vi "Flush ByteArray.vi"(8 "error in":errorcluster, 11 "Buffer":refnum<data-value>) -> (0 "error out":errorcluster, 2 "bytes":u8[](array[numeric]) format="%02x", 3 "Buffer":refnum<data-value>)   [LabVIEW 2013, in "ByteBuffer.lvclass"]
doc: "This VI returns data from the ring buffer starting from the oldest data and ending with the newest.\n\nThe data is duplicated at the output so this VI allocates new place in the memory for the output."
uses:
  ByteBuffer.lvclass
  VariantBuffer/VariantBuffer.lvclass
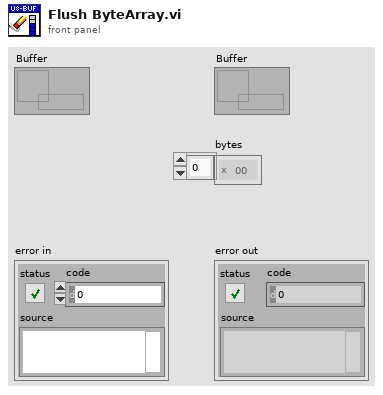
[diagram p1: front panel]
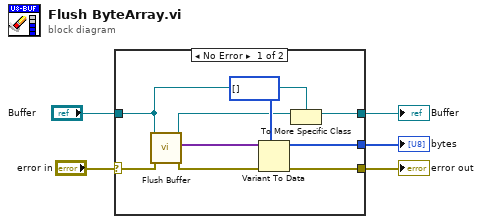
[diagram p0: block diagram]
diagram:
  n1 = case shown="No Error" "error in" {
    selector: "error in" -> [w14 w15]
    tunnel: "Buffer" -> [w6 w16]
    tunnel: [w7 w16] -> w4
    tunnel: [w12 w15] -> w1
    tunnel: [w9 _] -> w3
    frame No Error {
      n2 = call "Flush Buffer.vi"("error in"=w14, "Buffer in"=w6) -> ("error out"=w13:errorcluster, "elements"=w11:variant[], "Buffer"=w8:refnum<data-value>)  [unwired: 7 in]
      n3 = Variant To Data(error in=w13, type=u8[] [] ("bytes"), Variant=w11) -> (data=w9:u8[], error out=w12:errorcluster)
      n4 = To More Specific Class(target class=w6, reference=w8) -> (specific class reference=w7:refnum<data-value>)  [unwired: 1 in, 1 out]
    }
    frame Error {
    }
  }
  "error out" <- w1
  "Buffer" <- w4
  "bytes" <- w3
